vi "P2.vi"() -> ()   [LabVIEW 2018]
panel:
  in  "Image Type":T1 items=["Grayscale (U8)", "Grayscale (I16)", "Grayscale (SGL)", "Complex (CSG)", "RGB (U32)", "HSL (U32)", "RGB (U64)", "Grayscale (U16)"]
  in  "error in (no error)":errorcluster
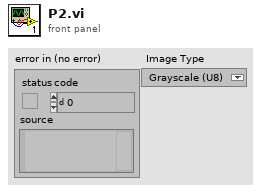
[diagram p1: front panel]
types:
  T1 = typedef "Image Type" = u32
  T2 = typedef "IMAQ Image.ctl" = refnum<image>
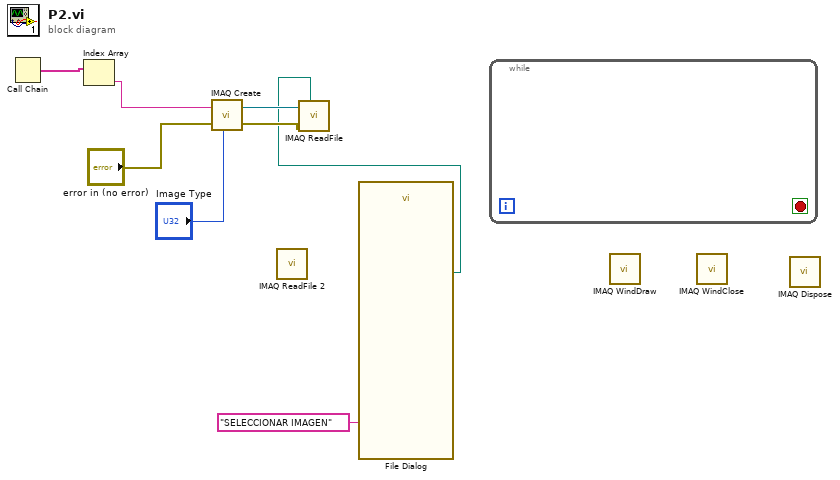
[diagram p0: block diagram]
diagram:
  n1 = Call Chain() -> (call chain=w7:string[])
  n2 = Index Array(array=w7) -> (element=w6:string)  [unwired: 1 in]
  n3 = call "IMAQ Create"("Image Name"=w6, "Image Type"="Image Type", "error in (no error)"="error in (no error)") -> ("New Image"=w5:T2, "error out"=w4:errorcluster)  [unwired: 2 in]
  n4 = call "IMAQ ReadFile 2"() -> ()  [unwired: 7 in, 5 out]
  n5 = call "File Dialog"("prompt"="SELECCIONAR IMAGEN") -> ("selected path"=w2:path)  [unwired: 11 in, 3 out]
  n6 = call <userlib>:"IMAQ ReadFile.vi"("File Path"=w2, "error in (no error)"=w4, "Image"=w5) -> ()  [unwired: 4 in, 5 out]
  n7 = while {
    stop <- _ stop-if-true
  }
  n8 = call "IMAQ WindDraw"() -> ()  [unwired: 10 in, 2 out]
  n9 = call "IMAQ WindClose"() -> ()  [unwired: 6 in, 1 out]
  n10 = call "IMAQ Dispose"() -> ()  [unwired: 6 in, 1 out]
